vi "checkSharedEnum.vi"(8 "error in (no error)":errorcluster, 9 "basicType":string, 10 "name":string, 11 "Topic in":refnum<class "Topic.lvclass">) -> (0 "error out":errorcluster, 1 "basicTypeUpdated":string, 2 "nameDup":string, 3 "Topic out":refnum<class "Topic.lvclass">)   [LabVIEW 2018, in "Topic.lvclass"]
doc: "Check the shared enum type and replace the original input data type if the shared enum is found."
uses:
  Topic.lvclass
  <vilib>/Utility/config.llb/NI_LVConfig.lvlib
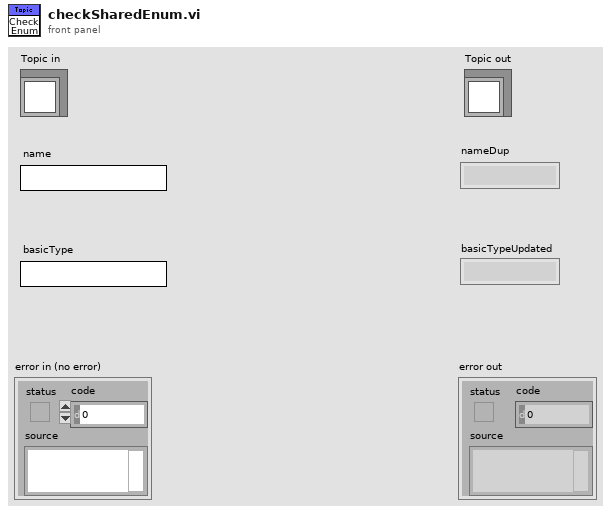
[diagram p1: front panel]
types:
  T1 = typedef "NI_LVConfig.lvlib/Config Data RefNum.ctl" = refnum<k1>
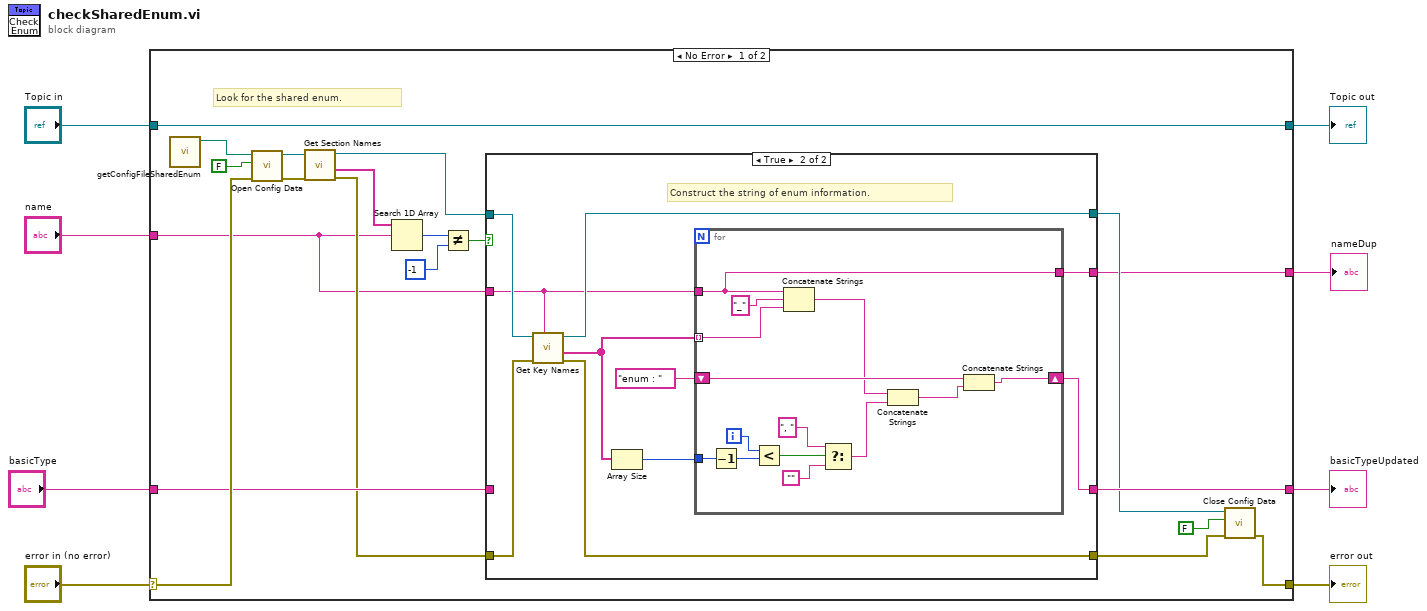
[diagram p0: block diagram]
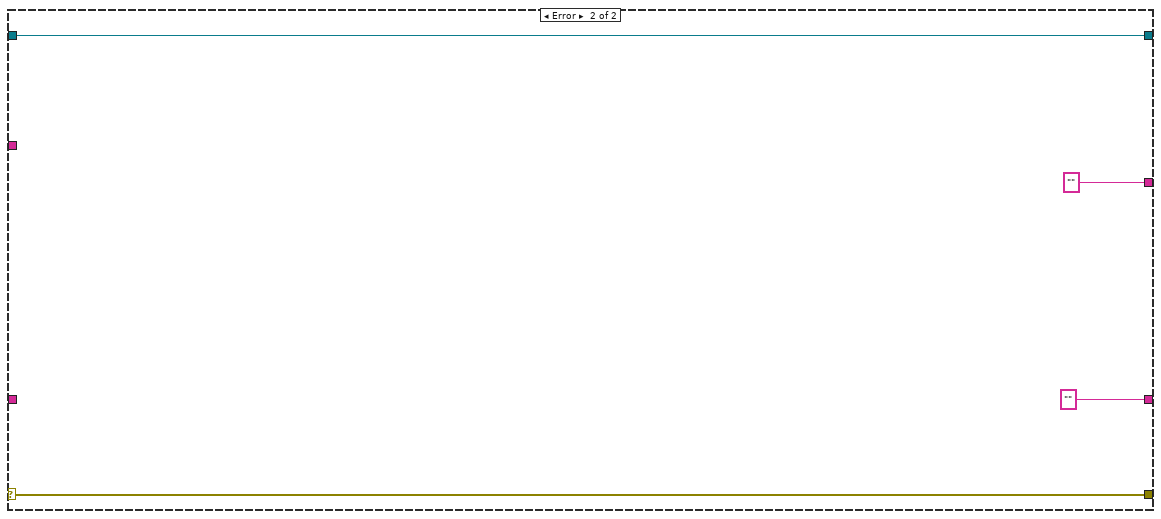
[diagram p3: hidden frame]
diagram:
  n1 = case shown="No Error" "error in (no error)" {
    selector: "error in (no error)" -> [w24 w60]
    tunnel: [w22 w60] -> w7
    tunnel: [w28 w59] -> w5
    tunnel: "Topic in" -> [w28 w59]
    tunnel: "name" -> [w13 _]
    tunnel: "basicType" -> [w18 _]
    tunnel: [w17 "" ("basicType")] -> w2
    tunnel: [w9 "" ("name")] -> w1
    frame No Error {
      # "Look for the shared enum."
      n2 = call "getConfigFileSharedEnum.vi"() -> ("configFileSharedEnum"=w27:path)  [unwired: 11 in]
      n3 = call <vilib>:"Open Config Data.vi"("error in (no error)"=w24, "create file if necessary (T)"=FALSE, "configuration file path"=w27) -> ("error out"=w25:errorcluster, "refnum"=w26:T1)  [unwired: 6 in, 1 out]
      n4 = call <vilib>:"Get Section Names.vi"("error in (no error)"=w25, "refnum"=w26) -> ("error out"=w16:errorcluster, "section names"=w23:string[], "refnum out"=w14:T1)  [unwired: 7 in]
      n5 = Search 1D Array(1D array=w23, element=w13) -> (index of element=w21:i32)  [unwired: 1 in]
      n6 = Not Equal?(x=w21, y=-1) -> (x != y?=w19:bool)
      n7 = case shown="True" w19 {
        tunnel: [w32 w37] -> w17
        tunnel: w18 -> [w32 _]
        tunnel: w16 -> [w31 w42]
        tunnel: [w31 w41] -> w15
        tunnel: w14 -> [w30 w40]
        tunnel: w13 -> [w29 w34]
        tunnel: [w30 w39] -> w12
        tunnel: [w29 w33] -> w9
        frame False {
        }
        frame True {
          # "Construct the string of enum information."
          n8 = call <vilib>:"Get Key Names.vi"("section"=w34, "error in (no error)"=w42, "refnum"=w40) -> ("error out"=w41:errorcluster, "key names"=w36:string[], "refnum out"=w39:T1)  [unwired: 5 in, 1 out]
          n9 = Array Size(array=w36) -> (size(s)=w35:i32)
          n10 = for {
            tunnel: w36 -> [w45] mode=indexing
            shift-right: [w47] -> w37
            shift-left: "enum : " -> [w49]
            tunnel: w35 -> [w56]
            tunnel: w34 -> [w43]
            tunnel: [w43] -> w33
            i -> [w54]
            n11 = Decrement(x=w56) -> (x-1=w55:i32)
            n12 = Less?(x=w54, y=w55) -> (x < y?=w53:bool)
            n13 = Concatenate Strings(w43, "_", w45) -> (w44:string)
            n14 = Select(t=", ", s=w53, f="") -> (s? t:f=w50:string)
            n15 = Concatenate Strings(w44, w50) -> (w48:string)
            n16 = Concatenate Strings(w49, w48) -> (w47:string)
          }
        }
      }
      n17 = call <vilib>:"Close Config Data.vi"("error in (no error)"=w15, "write file if changed (T)"=FALSE, "refnum"=w12) -> ("error out"=w22:errorcluster)  [unwired: 7 in, 1 out]
    }
    frame Error {
    }
  }
  "error out" <- w7
  "Topic out" <- w5
  "basicTypeUpdated" <- w2
  "nameDup" <- w1
